vi "Update DebugTools Project.vi"(7 "CD Folder Path":string, 8 "error in":errorcluster, 9 "DebugTools Project Path":path, 10 "CD Name":string, 11 "Project path":path) -> (0 "error out":errorcluster)   [LabVIEW 2026, in "NIVS_CDEW_MetaDataObj.lvclass"]
uses:
  NIVS_CDEW_MetaDataObj.lvclass
  NIVS_CDEW_MetaDataObj.lvclass/NIVS_CDEW_MetaDataObj.ctl
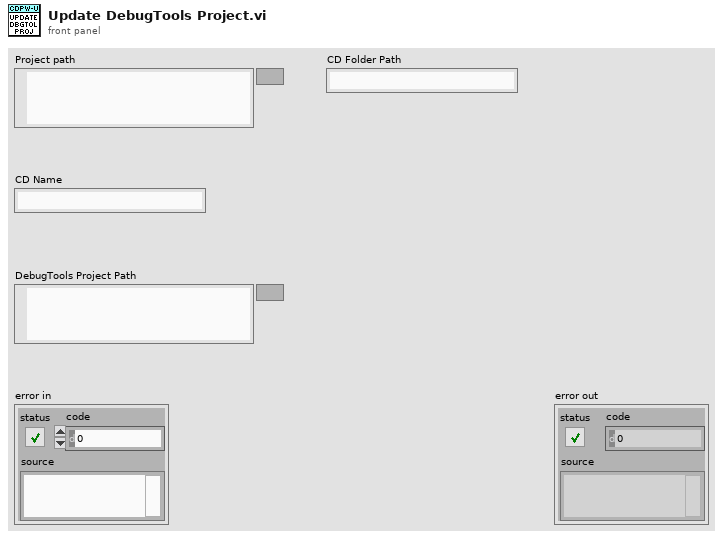
[diagram p1: front panel]
types:
  T1 = enum16{"open", "replace", "create", "open or create", "replace or create", "replace or create with confirmation"}
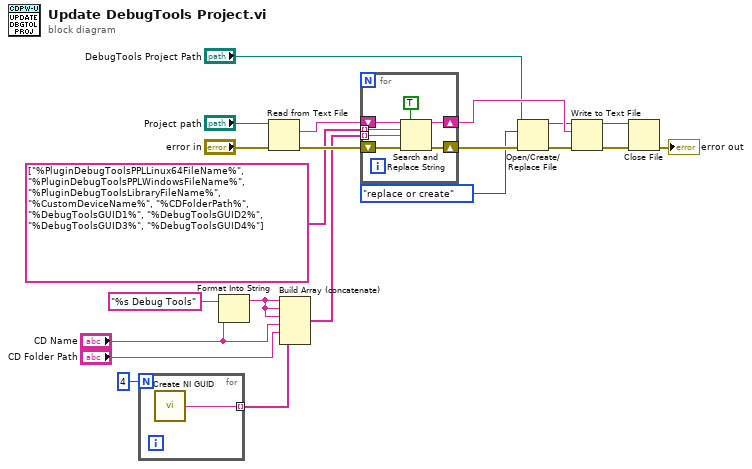
[diagram p0: block diagram]
diagram:
  n1 = for {
    N: 4 -> [_]
    tunnel: [w22] -> w1 mode=indexing
    n2 = call <vilib>:"Create NI GUID.vi"() -> ("NI GUID"=w22:string)
  }
  n3 = Format Into String(format string="%s Debug Tools" ("initial string"), "CD Name") -> (resulting string=w4:string)  [unwired: 2 in, 1 out]
  n4 = Read from Text File(file (use dialog)="Project path", error in="error in") -> (text=w16:string, error out=w19:errorcluster)  [unwired: 2 in, 2 out]
  n5 = Build Array (concatenate)(w4, w4, w4, "CD Name", "CD Folder Path", w1) -> (w14:string[])
  n6 = for {
    shift-right: [w28] -> w20
    shift-left: w19 -> [w27]
    shift-right: [w23] -> w13
    shift-left: w16 -> [w26]
    tunnel: string[] ["%PluginDebugToolsPPLLinux64FileName%", "%PluginDebugToolsPPLWindowsFileName%", "%PluginDebugToolsLibraryFileName%", "%CustomDeviceName%", "%CDFolderPath%", "%DebugToolsGUID1%", "%DebugToolsGUID2%", "%DebugToolsGUID3%", "%DebugToolsGUID4%"] -> [w25] mode=indexing
    tunnel: w14 -> [w24] mode=indexing
    n7 = Search and Replace String(replace all?=TRUE ("replace all? (F)"), input string=w26, search string=w25, replace string=w24, error in=w27) -> (result string=w23:string, error out=w28:errorcluster)  [unwired: 3 in, 2 out]
  }
  n8 = Open/Create/Replace File(file path (use dialog)="DebugTools Project Path", error in=w20, operation (0:open)=T1."replace or create") -> (refnum out=w11:refnum<file>, error out=w10:errorcluster)  [unwired: 3 in, 1 out]
  n9 = Write to Text File(file (use dialog)=w11, text=w13, error in=w10) -> (refnum out=w9:refnum<file>, error out=w8:errorcluster)  [unwired: 1 in, 1 out]
  n10 = Close File(refnum=w9, error in=w8) -> (error out=→"error out":errorcluster)  [unwired: 1 out]
